vi "EFMC-5.vi"(11 "数组输入":u8[](array[numeric])) -> (2 "修正值":T1, 3 "传感器信号":cluster{"陀螺温度":i16, "加计温度":i16})   [LabVIEW 2012]
uses:
  index-i16.vi
  XX-I16.vi
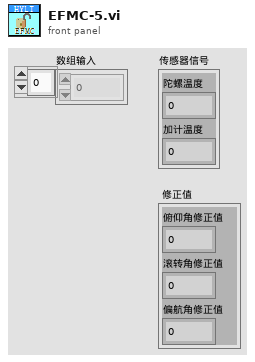
[diagram p1: front panel]
types:
  T1 = cluster{"俯仰角修正值":i16, "滚转角修正值":i16, "偏航角修正值":i16}
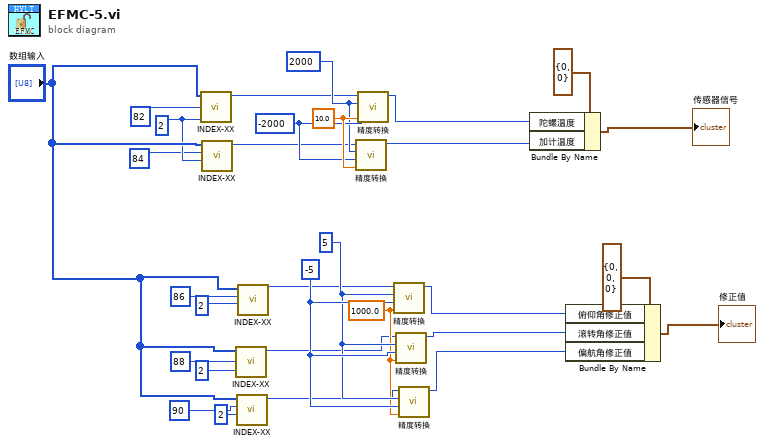
[diagram p0: block diagram]
diagram:
  w25 = i16 -5 ("下限")
  w24 = i16 5 ("上限")
  w19 = i16 -2000 ("下限")
  w18 = i16 2000 ("上限")
  w23 = 1000.0 ("单位")
  w20 = 10.0 ("单位")
  w17 = 2 ("长度")
  n1 = call-poly "INDEX-XX.vi"("长度"=w17, "索引"=82, "数组"="数组输入") -> ("数值输出"=w4:i16)  [unwired: 8 in]
  n2 = call-poly "INDEX-XX.vi"("长度"=w17, "索引"=84, "数组"="数组输入") -> ("数值输出"=w2:i16)  [unwired: 8 in]
  n3 = call-poly "INDEX-XX.vi"("长度"=2, "索引"=88, "数组"="数组输入") -> ("数值输出"=w10:i16)  [unwired: 8 in]
  n4 = call-poly "INDEX-XX.vi"("长度"=2, "索引"=90, "数组"="数组输入") -> ("数值输出"=w9:i16)  [unwired: 8 in]
  n5 = call-poly "INDEX-XX.vi"("长度"=2, "索引"=86, "数组"="数组输入") -> ("数值输出"=w12:i16)  [unwired: 8 in]
  n6 = call-poly "精度转换.vi"("单位"=w20, "下限"=w19, "上限"=w18, "数值输入"=w2) -> ("输出"=w1:i16)  [unwired: 7 in]
  n7 = call-poly "精度转换.vi"("单位"=w20, "下限"=w19, "上限"=w18, "数值输入"=w4) -> ("输出"=w3:i16)  [unwired: 7 in]
  n8 = call-poly "精度转换.vi"("单位"=w23, "下限"=w25, "上限"=w24, "数值输入"=w12) -> ("输出"=w11:i16)  [unwired: 7 in]
  n9 = call-poly "精度转换.vi"("单位"=w23, "下限"=w25, "上限"=w24, "数值输入"=w10) -> ("输出"=w8:i16)  [unwired: 7 in]
  n10 = call-poly "精度转换.vi"("单位"=w23, "下限"=w25, "上限"=w24, "数值输入"=w9) -> ("输出"=w7:i16)  [unwired: 7 in]
  n11 = Bundle By Name(cluster=cluster{"陀螺温度":i16, "加计温度":i16} {"陀螺温度"=0, "加计温度"=0} ("传感器信号 3"), "陀螺温度"=w3, "加计温度"=w1) -> (→"传感器信号":cluster{"陀螺温度":i16, "加计温度":i16})
  n12 = Bundle By Name(cluster=T1 {"俯仰角修正值"=0, "滚转角修正值"=0, "偏航角修正值"=0} ("修正值"), "俯仰角修正值"=w11, "滚转角修正值"=w8, "偏航角修正值"=w7) -> (→"修正值":T1)
